vi "DO Kmembrane.vi"(11 "Temperature (C)":dbl format="%.2f") -> (3 "Kmembrane":dbl format="%.2f")   [LabVIEW 2012]
panel:
  in  "Membrane Coefficient":dbl=0.05 format="%.2f"
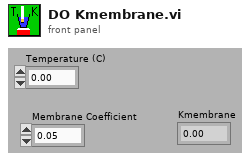
[diagram p1: front panel]
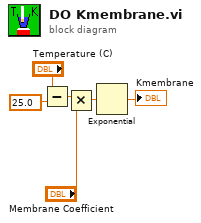
[diagram p0: block diagram]
diagram:
  n1 = Subtract(x="Temperature (C)", y=25.0) -> (x-y=w5:dbl)
  n2 = Multiply(x=w5, y="Membrane Coefficient") -> (x*y=w3:dbl)
  n3 = Exponential(1:w3) -> (0:→"Kmembrane":dbl)
